vi "IkiOpen.vi"(6 "error in (no error)":errorcluster, 9 "Iki Name":string) -> (0 "error out":errorcluster, 3 "connection ID":refnum<k5>)   [LabVIEW 2009]
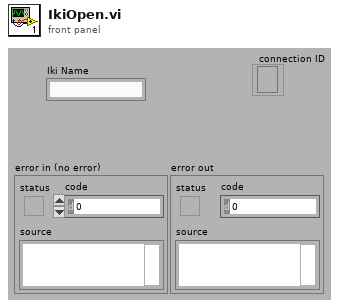
[diagram p1: front panel]
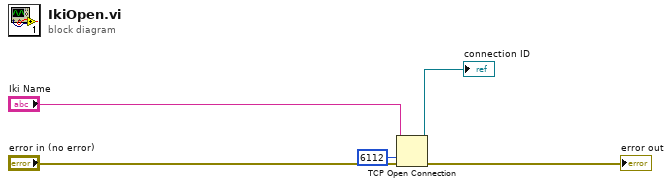
[diagram p0: block diagram]
diagram:
  n1 = TCP Open Connection(address="Iki Name", remote port or service name=u16 6112 ("port distant"), error in (no error)="error in (no error)") -> (connection ID=→"connection ID":refnum<k5>, error out=→"error out":errorcluster)  [unwired: 2 in]
